vi "JL_Verify Last Tone Played.vi"(0 "GEA2 Reference In":refnum<k24>, 1 "Verify Index?":bool, 2 "Verify Tune?":bool=TRUE, 7 "Expected Tone":T1, 9 "Expected Index":u8, 11 "Error In":errorcluster, 12 "Low Level Tries":u8=20 min=1) -> (4 "GEA2 Reference Out":refnum<k24>, 6 "Pass/Fail":bool, 8 "Report Text":string, 10 "Index":u8, 15 "Error Out":errorcluster)   [LabVIEW 2016]
uses:
  Common/Type Defs/JL_Tones.ctl
  Q:/Common/DLLs/GEA3/GeaCommunication.dll
  Common/DLLs/GEA3/GeaCommunication.dll
  Common/LabVIEW GEA2 Toolkit/LabVIEW_GEA2_Toolkit.lvlibp/type defs/Source_Destination.ctl
  Common/LabVIEW GEA2 Toolkit/LabVIEW_GEA2_Toolkit.lvlibp/type defs/ERD Read Data In.ctl
  Common/LabVIEW GEA2 Toolkit/LabVIEW_GEA2_Toolkit.lvlibp/type defs/Data Type.ctl
  Common/LabVIEW GEA2 Toolkit/LabVIEW_GEA2_Toolkit.lvlibp
panel:
  in  "Standalone?":bool
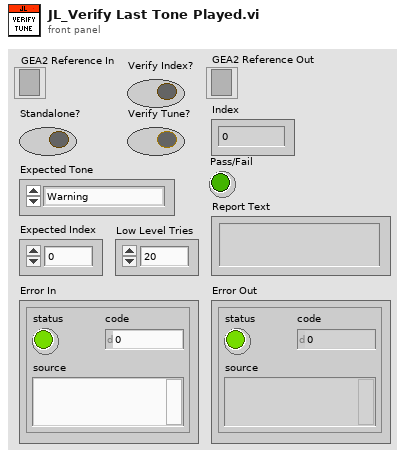
[diagram p1: front panel]
types:
  T1 = typedef "JL_Tones.ctl" = enum16{"Warning", "PowerUp", "PowerDown", "IncreaseSound", "DecreaseSound", "Ok", "OkVolumeKey", "Unavailable", "KnobTurn", "Notification1", "Notification2", "Notification3", "NotificationIntro", "NotificationEnd", "FeatureOn", "FeatureOff", "HoldOn", "HoldOnVolumeKey", "HoldOff", "Max", "None"}
  T2 = typedef "LabVIEW_GEA2_Toolkit.lvlibp/ERD Read Data In.ctl" = cluster{"ERD Number":u16, "Data Type":T3}
  T3 = typedef "LabVIEW_GEA2_Toolkit.lvlibp/Data Type.ctl" = enum16{"string", "boolean", "uint8_t", "uint16_t", "uint32_t", "uint64_t", "int8_t", "int16_t", "int32_t", "int64_t"}
  T4 = typedef "LabVIEW_GEA2_Toolkit.lvlibp/Source_Destination.ctl" = cluster{"Source":u8, "Destination":u8}
  T5 = typedef "LabVIEW_GEA2_Toolkit.lvlibp/ERD Read Data Out.ctl" = cluster{"ERD Number":u16, "Data":string}
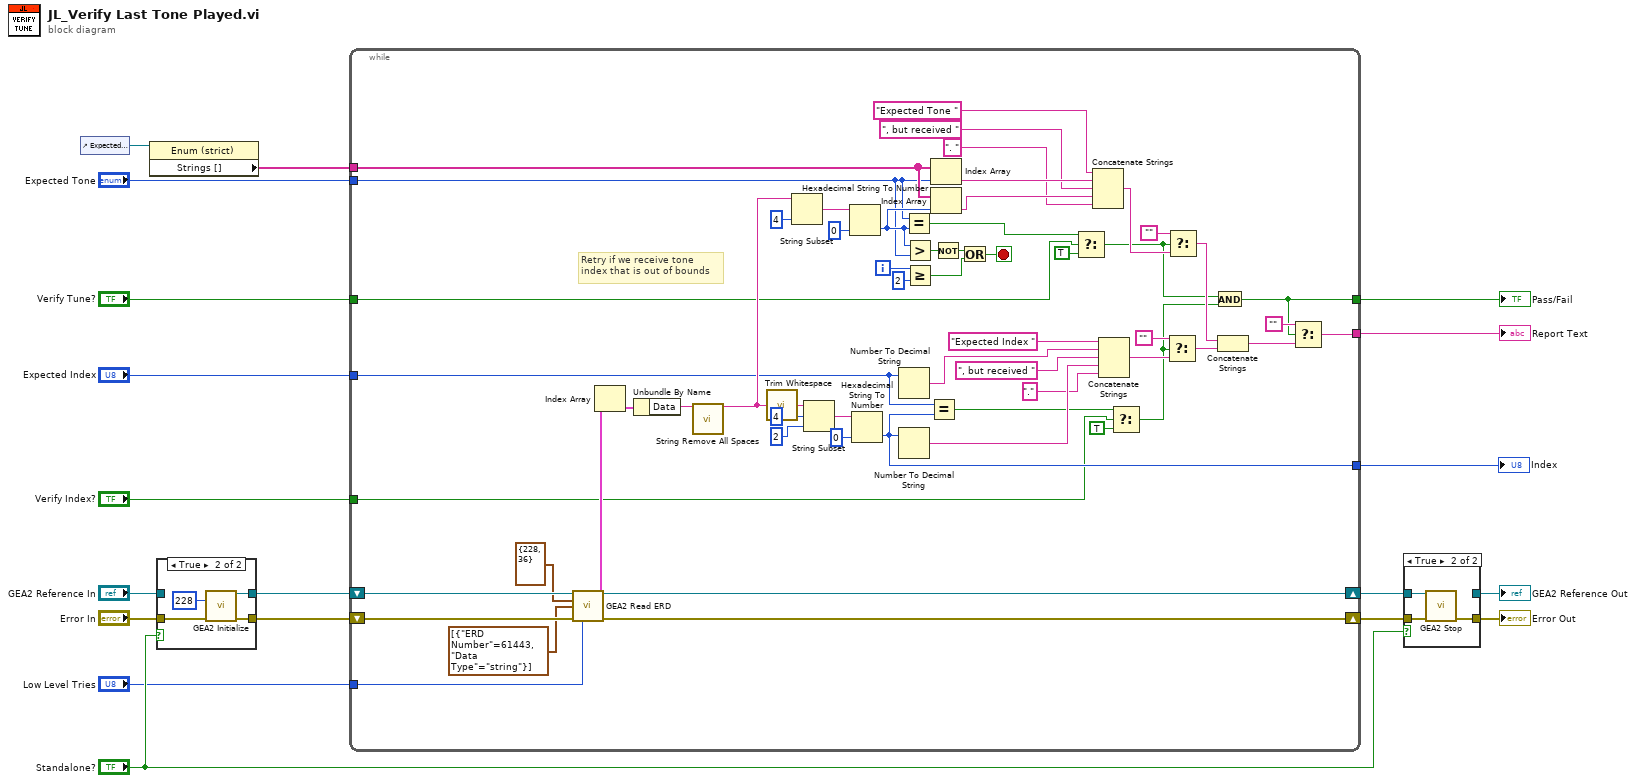
[diagram p0: block diagram]
diagram:
  n1 = control-ref of="Expected Tone"() -> (w1:refnum<vi>)
  n2 = property class="Enum (strict)"(reference=w1) -> ("Strings []"=w9:string[])  [unwired: 1 in, 2 out]
  n3 = case shown="True" "Standalone?" {
    tunnel: "Error In" -> [w21 w25]
    tunnel: [w21 w24] -> w15
    tunnel: [w20 w23] -> w16
    tunnel: "GEA2 Reference In" -> [w20 _]
    frame False {
    }
    frame True {
      n4 = call "GEA2 Initialize.vi"("Source Address"=u8 228, "error in"=w25) -> ("GEA2 Reference Out"=w23:refnum<k24>, "error out"=w24:errorcluster)  [unwired: 11 in, 1 out]
    }
  }
  n5 = while {
    tunnel: [w74] -> w10
    tunnel: "Expected Tone" -> [w34]
    tunnel: w9 -> [w70]
    tunnel: [w58] -> w7
    tunnel: "Expected Index" -> [w57]
    tunnel: "Verify Index?" -> [w36]
    shift-right: [w79] -> w14
    shift-left: w16 -> [w83]
    shift-right: [w78] -> w13
    shift-left: w15 -> [w82]
    tunnel: "Verify Tune?" -> [w41]
    tunnel: [w59] -> w8
    tunnel: "Low Level Tries" -> [w27]
    i -> [w32]
    stop <- w30 stop-if-true
    # "Retry if we receive tone\nindex that is out of bounds"
    n6 = call "GEA2 Read ERD.vi"("GEA2 Reference In"=w83, "GEA Inputs"=T4 {"Source"=228, "Destination"=36}, "Read ERD List"=T2[] [{"ERD Number"=61443, "Data Type"=enum."string"}], "Error In"=w82, "Low Level Tries"=w27) -> ("GEA2 Reference Out"=w79:refnum<k24>, "ERD Data Out"=w77:T5[], "Error Out"=w78:errorcluster)  [unwired: 7 in, 1 out]
    n7 = Index Array(array=w77) -> (element=w76:T5)  [unwired: 1 in]
    n8 = Unbundle By Name(w76) -> ("Data"=w68:string)
    n9 = call "String Remove All Spaces.vi"("Input String"=w68) -> ("Spaces Removed"=w67:string)  [unwired: 13 in, 1 out]
    n10 = call <vilib>:"Trim Whitespace.vi"("string"=w67) -> ("trimmed string"=w26:string)  [unwired: 1 in]
    n11 = String Subset(string=w67, length (rest)=4 ("length (rest)")) -> (substring=w64:string)  [unwired: 1 in]
    n12 = String Subset(string=w26, offset (0)=4, length (rest)=2 ("length (rest)")) -> (substring=w63:string)
    n13 = Hexadecimal String To Number(string=w64, default (0uL)=u16 0 ("default (0 I32)")) -> (number=w35:u16)  [unwired: 1 in, 1 out]
    n14 = Hexadecimal String To Number(string=w63, default (0uL)=u8 0 ("default (0 U32)")) -> (number=w58:u8)  [unwired: 1 in, 1 out]
    n15 = Number To Decimal String(number=w57) -> (decimal integer string=w55:string)  [unwired: 1 in]
    n16 = Number To Decimal String(number=w58) -> (decimal integer string=w53:string)  [unwired: 1 in]
    n17 = Equal?(x=w34, y=w35) -> (x = y?=w43:bool)
    n18 = Greater?(x=w35, y=w34) -> (0:w29:bool)
    n19 = Greater Or Equal?(x=w32, y=2) -> (x >= y?=w33:bool)
    n20 = Equal?(x=w57, y=w58) -> (x = y?=w38:bool)
    n21 = Index Array(array=w70, index=w34) -> (element=w71:string)
    n22 = Index Array(array=w70, index=w35) -> (element=w69:string)
    n23 = Not(x=w29) -> (.not. x?=w28:bool)
    n24 = Or(x=w28, y=w33) -> (x .or. y?=w30:bool)
    n25 = Select(t=w43, s=w41, f=TRUE) -> (s? t:f=w42:bool)
    n26 = Concatenate Strings("Expected Tone " ("string"), w71, ", but received " ("string"), w69, ". " ("string")) -> (w50:string)
    n27 = Concatenate Strings("Expected Index " ("string"), w55, ", but received " ("string"), w53, "." ("string")) -> (w46:string)
    n28 = Select(t=w38, s=w36, f=TRUE) -> (s? t:f=w37:bool)
    n29 = Select(t="", s=w37, f=w46) -> (s? t:f=w45:string)
    n30 = Select(t="", s=w42, f=w50) -> (s? t:f=w49:string)
    n31 = And(x=w42, y=w37) -> (x .and. y?=w59:bool)
    n32 = Concatenate Strings(w49, w45) -> (w48:string)
    n33 = Select(t="", s=w59, f=w48) -> (s? t:f=w74:string)
  }
  "Pass/Fail" <- w8
  "Report Text" <- w10
  "Index" <- w7
  n34 = case shown="True" "Standalone?" {
    tunnel: [w84 w88] -> w11
    tunnel: w14 -> [w85 w87]
    tunnel: w13 -> [w84 w86]
    tunnel: [w85 _] -> w12
    frame False {
    }
    frame True {
      n35 = call "GEA2 Stop.vi"("GEA2 Reference In"=w87, "Error In"=w86) -> ("Error Out"=w88:errorcluster)  [unwired: 13 in]
    }
  }
  "Error Out" <- w11
  "GEA2 Reference Out" <- w12
